vi "ref_Elbow_SEA_Oriental_position_control_frequency_lys_pwm.vi"() -> ()   [LabVIEW 2014]
uses:
  <vilib>/rvi/FXPMathLib/FxpSub/XNode/nifxpmath_Sub.xnode
  <vilib>/rvi/FXPMathLib/sim/FxpSim.dll
  <vilib>/rvi/FXPMathLib/FxpMul/XNode/nifxpmath_Multiplier.xnode
  <vilib>/rvi/FXPMathLib/FxpAdd/XNode/nifxpmath_Add.xnode
  <vilib>/eio/EIONode/EIONode.xnode
  <vilib>/rvi/eio/common/nirviEmuTemplateMethod_errors.vi
  <vilib>/rvi/FXPMathLib/FxpSinAndCos/subVIs/nifxpmath_SinAndCos_SimConfig.ctl
  <vilib>/rvi/FXPMathLib/FxpSinAndCos/simVIs/DllFxpSinAndCosTemp_sub.vi
  <vilib>/rvi/FXPMathLib/FxpSinAndCos/XNode/nifxpmath_SinAndCos.xnode
  <vilib>/rvi/Analysis/measure/butterworth/XNode/niFpgaButterworthFilter.xnode
  <vilib>/rvi/DataTransferAndStorage/Container/XNode/niFpgaContainer.xnode
  <vilib>/rvi/interface/RandomDataEmulation/nirviRandomDataFpgaMultiElementTemplate.vi
panel:
  in  "pwm method":i32
  out "tri_wave time (s)":fxp<+,64,32>
  out "vb_ pwm":fxp<+/-,21,6> format="%.21g"
  out "vb_ori":fxp<+/-,20,5> format="%.21g"
  out "va_pwm":fxp<+/-,21,6> format="%.21g"
  out "va_ori":fxp<+/-,20,5> format="%.21g"
  out "pwm_signal 2":fxp<+/-,20,5>
  in  "PWM ON":bool
  out "pwm_signal":fxp<+/-,13,6>
  out "tri_wave Ts (s)":fxp<+,37,17>=0.0009765625
  in  "Sin_magnitude_b(mm)":fxp<+/-,11,8>
  in  "Sin_offset_b (mm)":fxp<+/-,12,8>
  out "sin_signal":fxp<+/-,20,5>
  in  "Sin wave frenqueny (Hz)":fxp<+,18,3>
  out "tri_wave":fxp<+/-,64,32>
  in  "tri_wave frequency (Hz)":fxp<+,36,20>
  in  "Vdc":fxp<+,12,5>
  in  "scaled coefficients_dFb_PID":i32[](array[numeric])=[1067016412, 3362706]
  in  "Coe Ini":bool
  out "chirp_signal":fxp<+/-,36,11>
  out "frequency (Hz)":fxp<+,24,9>
  in  "Sin wave amplitude (mm)":fxp<+,20,11>
  in  "Db_step (mm)":fxp<+/-,36,11>
  in  "Step/Chirp":bool
  in  "initial frenqueny (Hz)":fxp<+,20,5>
  in  "target frenqueny (Hz)":fxp<+,23,8>
  in  "target time (s)":fxp<+,24,9>
  out "Sin wave time (s)":fxp<+,64,32>
  out "vb_b":fxp<+/-,20,5> format="%.21g"
  out "va_b":fxp<+/-,20,5> format="%.21g"
  in  "Stop Motor_b":bool
  out "dFb_PID":fxp<+/-,25,15>
  in  "dF_PID_add":bool
  out "vd_b_F":fxp<+/-,20,5>
  out "vq_b_F":fxp<+/-,20,5> format="%.57g"
  out "rad(NrTheta)_b":fxp<+/-,33,18> format="%.21g"
  out "Db(mm)":fxp<+/-,22,7>
  in  "Encoder Reset_b":bool
  in  "Db_d_M_Tc (mSec)":u32 format="%#_6f"
  out "mt_omega":u32
  in  "mt0_omega":u32
  in  "Db_M_avg_Tc (uSec)":u32
  out "Encoder Position_b":i32
  out "Omega_b(M)":fxp<+/-,32,12>
  out "Db_d(M method)":fxp<+/-,25,10>
  out "Omega_b(M_avg)":fxp<+/-,32,12>
  out "Db_d(M_avg method)":fxp<+/-,25,10>
  in  "Method case":i32
  out "Db_d(mm/s)":fxp<+/-,25,10>
  out "Omega_b(rad/s)":fxp<+/-,32,12>
  out "Omega_b(T)":fxp<+/-,20,9>
  out "Db_d(T method)":fxp<+/-,25,10>
  in  "Friction comp_b":fxp<+/-,20,10>
  out "Dbr":fxp<+/-,36,11>
  out "Dbr_d":fxp<+/-,25,15>
  out "Dbt_i":fxp<+/-,34,18>
  out "Fb_PID":fxp<+/-,22,12>
  in  "Db_tolerance":fxp<+,32,9>=1.0
  out "Db_tilde":fxp<+/-,21,11>
  in  "Kpb":fxp<+,12,8>=0.375
  in  "Kib":fxp<+,27,10>
  in  "Kdb":fxp<+,26,2>
  in  "FF or not":bool
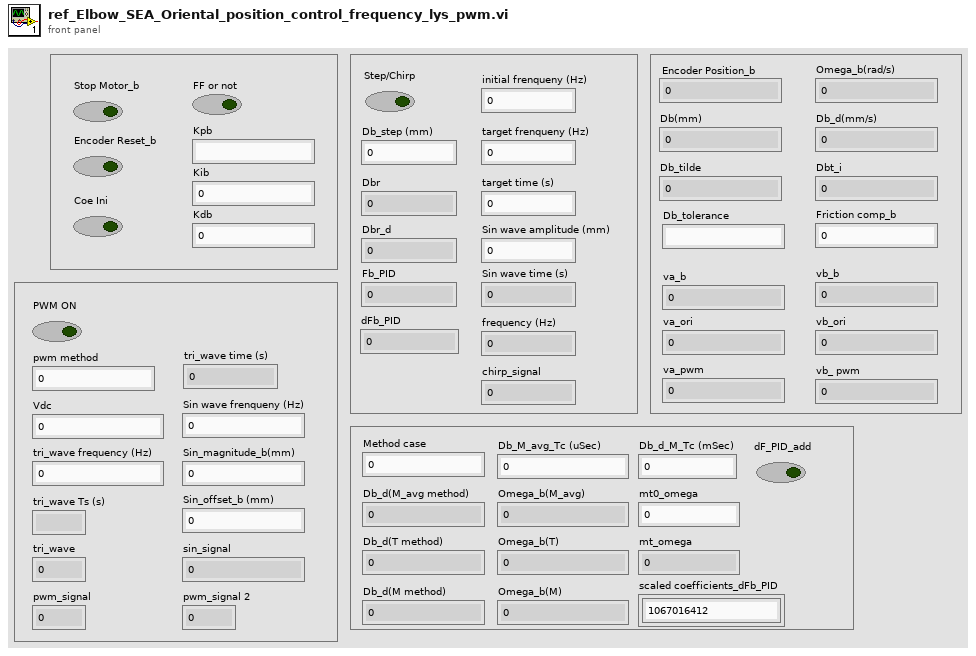
[diagram p1: front panel]
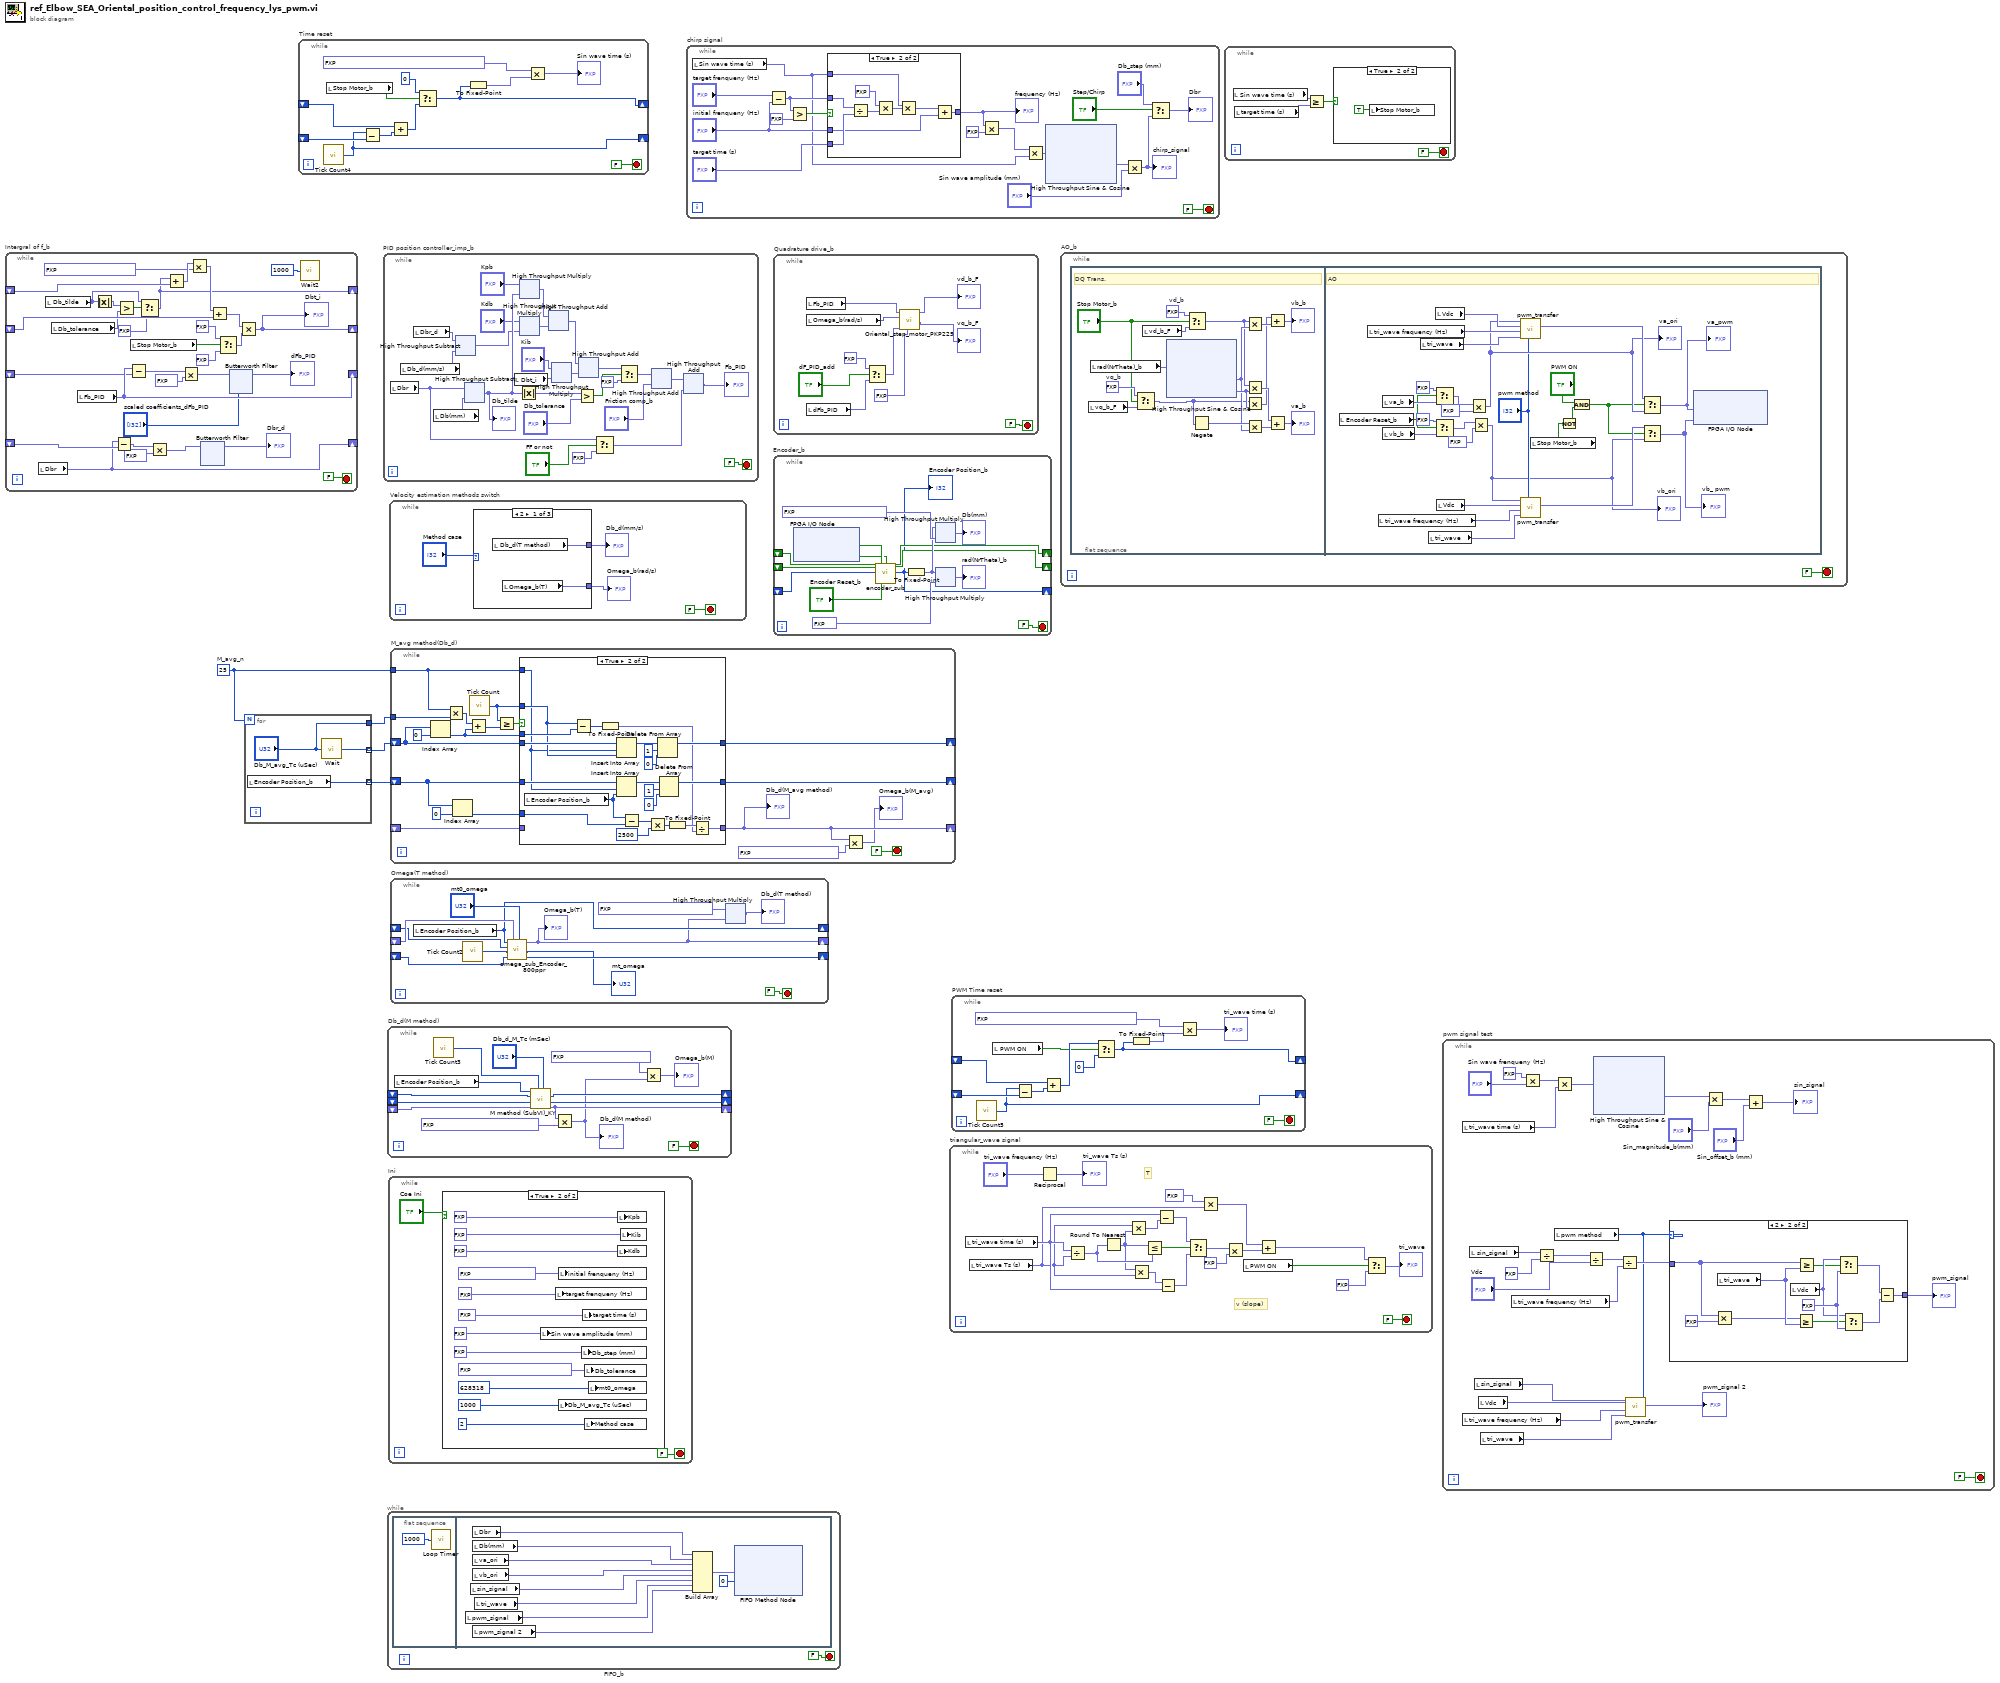
[diagram p0: block diagram]
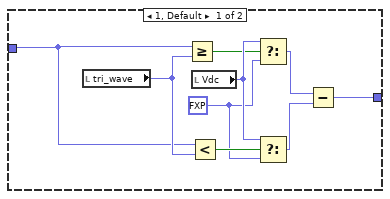
[diagram p2: hidden frame]
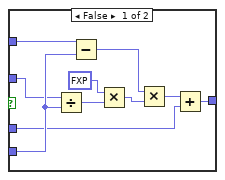
[diagram p5: hidden frame]
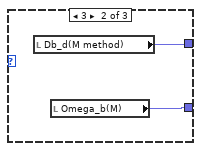
[diagram p7: hidden frame]
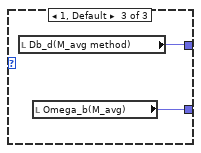
[diagram p8: hidden frame]
diagram:
  w2 = 25  # M_avg_n
  n1 = while "Intergral of f_b" {
    shift-right: [w24] -> _
    shift-left: _ -> [w25]
    shift-right: [w6] -> _
    shift-left: _ -> [w30]
    shift-right: [w20] -> _
    shift-left: _ -> [w18]
    shift-right: [w12] -> _
    shift-left: _ -> [w13]
    stop <- FALSE stop-if-true
    n2 = local read "Dbr"() -> (w12:fxp<+/-,36,11>)
    n3 = local read "Db_tilde"() -> (w26:fxp<+/-,21,11>)
    n4 = local read "Db_tolerance"() -> (w28:fxp<+,32,9>)
    n5 = local read "Fb_PID"() -> (w20:fxp<+/-,22,12>)
    n6 = Absolute Value(x=w26) -> (abs(x)=w29:fxp<+,21,11>)
    n7 = Subtract(x=w12, y=w13) -> (x-y=w15:fxp<+/-,37,12>)
    n8 = Greater?(x=w29, y=w28) -> (0:w27:bool)
    n9 = Subtract(x=w20, y=w18) -> (x-y=w19:fxp<+/-,23,13>)
    n10 = local read "Stop Motor_b"() -> (w32:bool)
    n11 = Select(t=w26, s=w27, f=fxp<+/-,21,11> 0.0) -> (s? t:f=w24:fxp<+/-,21,11>)
    n12 = Multiply(x=w15, y=fxp<+/-,24,11> 1000.0) -> (x*y=w14:fxp<+/-,25,15>)
    n13 = Add(x=w24, y=w25) -> (x+y=w34:fxp<+/-,22,12>)
    n14 = Multiply(x=w19, y=fxp<+,10,10> 1000.0) -> (x*y=w17:fxp<+/-,25,15>)
    n15 = Multiply(x=w34, y=fxp<+/-,30,12> 0.000499725341796875) -> (x*y=w31:fxp<+/-,25,15>)
    n16 = xnode "Butterworth Filter"("input data"=w14) -> ("output data"=→"Dbr_d":fxp<+/-,25,15>)  [unwired: 2 in]
    n17 = Add(x=w31, y=w30) -> (x+y=w9:fxp<+/-,32,16>)
    n18 = Select(t=fxp<+/-,2,2> 0.0, s=w32, f=fxp<+/-,2,2> 1.0) -> (s? t:f=w10:fxp<+/-,2,2>)
    n19 = xnode "Butterworth Filter"("input data"=w17, "scaled coefficients"="scaled coefficients_dFb_PID") -> ("output data"=→"dFb_PID":fxp<+/-,25,15>)  [unwired: 1 in]
    n20 = Multiply(x=w9, y=w10) -> (x*y=w6:fxp<+/-,34,18>)
    "Dbt_i" <- w6
    n21 = call "Wait2"("Count(uSec)"=u32 1000 ("Count(mSec)")) -> ()  [unwired: 1 out]
  }
  n22 = for {
    N: w2 -> [_]
    tunnel: [w55] -> w4 mode=indexing
    tunnel: [w53] -> w3 mode=indexing
    tunnel: ["Db_M_avg_Tc (uSec)"] -> w1
    n23 = local read "Encoder Position_b"() -> (w53:i32)
    n24 = call "Wait"("Count(uSec)"="Db_M_avg_Tc (uSec)") -> ("Tick Count(uSec)"=w55:u32)
  }
  n25 = while "Time reset" {
    shift-right: [w66] -> _
    shift-left: _ -> [w67]
    shift-right: [w59] -> _
    shift-left: _ -> [w61]
    stop <- FALSE stop-if-true
    n26 = call "Tick Count4"() -> ("Tick Count(uSec)"=w66:u32)
    n27 = local read "Stop Motor_b"() -> (w64:bool)
    n28 = Subtract(x=w66, y=w67) -> (x-y=w63:u32)
    n29 = Add(x=w61, y=w63) -> (x+y=w62:u32)
    n30 = Select(t=u32 0, s=w64, f=w62) -> (s? t:f=w59:u32)
    n31 = To Fixed-Point(number=w59) -> (fixed-point=w57:fxp<+,64,32>)  [unwired: 1 in]
    n32 = Multiply(x=fxp<+,20,-18> 1.0000003385357559e-06 ("y"), y=w57) -> (x*y=→"Sin wave time (s)":fxp<+,64,32>)
  }
  n33 = while "PID position controller_imp_b" {
    stop <- FALSE stop-if-true
    n34 = local read "Dbr"() -> (w69:fxp<+/-,36,11>)
    n35 = local read "Db_d(mm/s)"() -> (w76:fxp<+/-,25,10>)
    n36 = local read "Dbr_d"() -> (w75:fxp<+/-,25,15>)
    n37 = local read "Db(mm)"() -> (w87:fxp<+/-,22,7>)
    n38 = xnode "High Throughput Subtract"("x"=w75, "y"=w76) -> ("x-y"=w77:fxp<+/-,31,16>)
    n39 = xnode "High Throughput Subtract"("x"=w69, "y"=w87) -> ("x-y"=w89:fxp<+/-,21,11>)
    "Db_tilde" <- w89
    n40 = local read "Dbt_i"() -> (w85:fxp<+/-,34,18>)
    n41 = Absolute Value(x=w89) -> (abs(x)=w92:fxp<+,21,11>)
    n42 = xnode ("High Throughput Multiply")("x"="Kpb", "y"=w89) -> ("x*y"=w88:fxp<+/-,33,17>)
    n43 = xnode ("High Throughput Multiply")("x"="Kdb", "y"=w77) -> ("x*y"=w82:fxp<+/-,31,21>)
    n44 = xnode ("High Throughput Add")("x"=w88, "y"=w82) -> ("x+y"=w86:fxp<+/-,22,12>)
    n45 = xnode ("High Throughput Multiply")("x"="Kib", "y"=w85) -> ("x*y"=w84:fxp<+/-,31,14>)
    n46 = Greater?(x=w92, y="Db_tolerance") -> (0:w91:bool)
    n47 = xnode ("High Throughput Add")("x"=w86, "y"=w84) -> ("x+y"=w83:fxp<+/-,22,12>)
    n48 = Select(t=w69, s="FF or not", f=fxp<+/-,36,11> 0.0) -> (s? t:f=w71:fxp<+/-,36,11>)
    n49 = Select(t=w83, s=w91, f=fxp<+/-,20,10> 0.0) -> (s? t:f=w81:fxp<+/-,22,12>)
    n50 = xnode ("High Throughput Add")("x"=w81, "y"="Friction comp_b") -> ("x+y"=w73:fxp<+/-,22,12>)
    n51 = xnode ("High Throughput Add")("x"=w73, "y"=w71) -> ("x+y"=→"Fb_PID":fxp<+/-,22,12>)
  }
  n52 = while "Db_d(M method)" {
    shift-right: [w106] -> _
    shift-left: _ -> [w101]
    shift-right: [w105] -> _
    shift-left: _ -> [w100]
    shift-right: [w98] -> _
    shift-left: _ -> [w99]
    stop <- FALSE stop-if-true
    n53 = local read "Encoder Position_b"() -> (w102:i32)
    n54 = call "Tick Count3"() -> ("Tick Count(mSec)"=w103:u32)
    n55 = call "M method (SubVI)_KY.vi"("Tc (mSec)"="Db_d_M_Tc (mSec)", "Tick Count (mSec)"=w103, "Encoder velocity_pre (pulse/s)"=w99, "Shift Register in 2"=w100, "Shift Register in 1"=w101, "Encoder pulses"=w102) -> ("Encoder velocity (pulse/s)"=w98:fxp<+/-,64,32>, "Shift Register out 2"=w105:i32, "Shift Register out 1"=w106:u32)  [unwired: 3 in]
    n56 = Multiply(x=w98, y=fxp<+/-,20,-5> 0.002499997615814209) -> (x*y=w95:fxp<+/-,25,10>)
    "Db_d(M method)" <- w95
    n57 = Multiply(x=fxp<+/-,32,12> 3.1415929794311523, y=w95) -> (x*y=→"Omega_b(M)":fxp<+/-,32,12>)
  }
  n58 = while "FIFO_b" {
    stop <- FALSE stop-if-true
    n59 = flat-sequence {
      frame #0 {
        n60 = call "Loop Timer"("Count(uSec)"=u32 1000 ("Loop Period (usec)")) -> ()  [unwired: 1 out]
      }
      frame #1 {
        n61 = local read "pwm_signal"() -> (w113:fxp<+/-,13,6>)
        n62 = local read "sin_signal"() -> (w114:fxp<+/-,20,5>)
        n63 = local read "Dbr"() -> (w117:fxp<+/-,36,11>)
        n64 = local read "Db(mm)"() -> (w116:fxp<+/-,22,7>)
        n65 = local read "va_ori"() -> (w115:fxp<+/-,20,5>)
        n66 = local read "vb_ori"() -> (w120:fxp<+/-,20,5>)
        n67 = local read "pwm_signal 2"() -> (w119:fxp<+/-,20,5>)
        n68 = local read "tri_wave"() -> (w112:fxp<+/-,64,32>)
        n69 = Build Array(w117, w116, w115, w120, w114, w112, w113, w119) -> (w111:fxp<+/-,64,32>[])
        n70 = xnode ("FIFO Method Node")("Element"=w111, "Timeout"=0) -> ()  [unwired: 1 in, 2 out]
      }
    }
  }
  n71 = while "Ini" {
    stop <- FALSE stop-if-true
    n72 = case shown="True" "Coe Ini" {
      frame False {
      }
      frame True {
        n73 = local write "Sin wave amplitude (mm)"(fxp<+,20,11> 0.0 ("target frenqueny (Hz)")) -> ()
        n74 = local write "target frenqueny (Hz)"(fxp<+,23,8> 10.0 ("target frenqueny (Hz)")) -> ()
        n75 = local write "initial frenqueny (Hz)"(fxp<+,20,5> 0.100006103515625 ("initial frenqueny (Hz)")) -> ()
        n76 = local write "Db_M_avg_Tc (uSec)"(u32 1000 ("M_avg_Tc (uSec)")) -> ()
        n77 = local write "Db_step (mm)"(fxp<+/-,36,11> 0.0 ("target frenqueny (Hz)")) -> ()
        n78 = local write "target time (s)"(fxp<+,24,9> 120.0 ("target time (s)")) -> ()
        n79 = local write "Db_tolerance"(fxp<+,32,9> 0.10000002384185791) -> ()
        n80 = local write "Method case"(2 ("M_avg_Tc (uSec)")) -> ()
        n81 = local write "mt0_omega"(u32 628318 ("mt0_omega")) -> ()
        n82 = local write "Kpb"(fxp<+,11,7> 0.0) -> ()
        n83 = local write "Kdb"(fxp<+,26,2> 0.0) -> ()
        n84 = local write "Kib"(fxp<+,27,10> 0.0 ("Kiy 2")) -> ()
      }
    }
  }
  n85 = while "Velocity estimation methods switch" {
    stop <- FALSE stop-if-true
    n86 = case shown="2" "Method case" {
      tunnel: [w139 w141 w143] -> w136
      tunnel: [w140 w142 w144] -> w135
      frame 2 {
        n87 = local read "Db_d(T method)"() -> (w139:fxp<+/-,25,10>)
        n88 = local read "Omega_b(T)"() -> (w140:fxp<+/-,20,9>)
      }
      frame 3 {
        n89 = local read "Db_d(M method)"() -> (w141:fxp<+/-,25,10>)
        n90 = local read "Omega_b(M)"() -> (w142:fxp<+/-,32,12>)
      }
      frame 1, Default {
        n91 = local read "Db_d(M_avg method)"() -> (w143:fxp<+/-,25,10>)
        n92 = local read "Omega_b(M_avg)"() -> (w144:fxp<+/-,32,12>)
      }
    }
    "Db_d(mm/s)" <- w136
    "Omega_b(rad/s)" <- w135
  }
  n93 = while "M_avg method(Db_d)" {
    shift-right: [w155] -> _
    shift-left: w4 -> [w158]
    tunnel: w2 -> [w156]
    shift-right: [w153] -> _
    shift-left: w3 -> [w151]
    shift-right: [w146] -> _
    shift-left: _ -> [w149]
    tunnel: w1 -> [w148]
    stop <- FALSE stop-if-true
    n94 = Index Array(array=w158, index=0) -> (element=w154:u32)
    n95 = Multiply(x=w156, y=w148) -> (x*y=w161:u32)
    n96 = Index Array(array=w151, index=0) -> (element=w150:i32)
    n97 = Add(x=w161, y=w154) -> (x+y=w160:u32)
    n98 = call "Tick Count"() -> ("Tick Count(uSec)"=w157:u32)
    n99 = Greater Or Equal?(x=w157, y=w160) -> (x >= y?=w159:bool)
    n100 = case shown="True" w159 {
      tunnel: w158 -> [w166 w188]
      tunnel: w157 -> [_ w182]
      tunnel: w156 -> [_ w171]
      tunnel: [w166 w184] -> w155
      tunnel: w154 -> [_ w183]
      tunnel: w151 -> [w165 w172]
      tunnel: [w165 w170] -> w153
      tunnel: [w164 w169] -> w146
      tunnel: w150 -> [_ w167]
      tunnel: w149 -> [w164 _]
      frame False {
      }
      frame True {
        n101 = local read "Encoder Position_b"() -> (w176:i32)
        n102 = Subtract(x=w182, y=w183) -> (x-y=w181:u32)
        n103 = To Fixed-Point(number=w181) -> (fixed-point=w168:fxp<+,32,32>)  [unwired: 1 in]
        n104 = Insert Into Array(array=w188, index=w171, new element=w182) -> (w187:u32[])
        n105 = Insert Into Array(array=w172, index=w171, new element=w176) -> (w173:i32[])
        n106 = Subtract(x=w176, y=w167) -> (x-y=w177:i32)
        n107 = Multiply(x=w177, y=2500) -> (x*y=w179:i32)
        n108 = Delete From Array(array=w187, length=1, index=0) -> (array with subset deleted=w184:u32[])  [unwired: 1 out]
        n109 = Delete From Array(array=w173, length=1, index=0) -> (array with subset deleted=w170:i32[])  [unwired: 1 out]
        n110 = To Fixed-Point(number=w179) -> (fixed-point=w180:fxp<+/-,32,32>)  [unwired: 1 in]
        n111 = Divide(x=w180, y=w168) -> (x/y=w169:fxp<+/-,25,10>)
      }
    }
    "Db_d(M_avg method)" <- w146
    n112 = Multiply(x=w146, y=fxp<+/-,32,12> 3.1415929794311523 ("x")) -> (x*y=→"Omega_b(M_avg)":fxp<+/-,32,12>)
  }
  n113 = while "Omega(T method)" {
    shift-right: [w193] -> _
    shift-left: _ -> [w192]
    shift-right: [w199] -> _
    shift-left: _ -> [w194]
    shift-right: [w190] -> _
    shift-left: _ -> [w196]
    stop <- FALSE stop-if-true
    n114 = local read "Encoder Position_b"() -> (w193:i32)
    n115 = call "Tick Count2"() -> ("Tick Count(Ticks)"=w195:u32)
    n116 = call "omega_sub_Encoder_800ppr.vi"("mt0"="mt0_omega", "omega_pre"=w196, "ticks_m_pre"=w194, "ticks"=w195, "count_pre"=w192, "count"=w193) -> ("ticks_m"=w199:u32, "mt"=→"mt_omega":u32, "omega"=w190:fxp<+/-,20,9>)  [unwired: 3 in]
    "Omega_b(T)" <- w190
    n117 = xnode ("High Throughput Multiply")("x"=fxp<+/-,26,1> 0.3183099031448364, "y"=w190) -> ("x*y"=→"Db_d(T method)":fxp<+/-,24,9>)
  }
  n118 = while "chirp signal" {
    stop <- FALSE stop-if-true
    n119 = local read "Sin wave time (s)"() -> (w202:fxp<+,64,32>)
    n120 = Subtract(x="target frenqueny (Hz)", y="initial frenqueny (Hz)") -> (x-y=w203:fxp<+/-,24,9>)
    n121 = Greater?(x=w203, y=fxp<+/-,24,9> 0.0) -> (0:w206:bool)
    n122 = case shown="True" w206 {
      tunnel: [w227 w236] -> w211
      tunnel: "target time (s)" -> [w224 w235]
      tunnel: "initial frenqueny (Hz)" -> [w223 w234]
      tunnel: w202 -> [w226 w233]
      tunnel: w203 -> [w222 w232]
      frame False {
        n123 = Divide(x=w222, y=w224) -> (x/y=w221:fxp<+/-,24,9>)
        n124 = Subtract(x=w226, y=w224) -> (x-y=w225:fxp<+/-,24,9>)
        n125 = Multiply(x=fxp<+/-,24,9> 0.5, y=w221) -> (x*y=w220:fxp<+/-,23,10>)
        n126 = Multiply(x=w225, y=w220) -> (x*y=w228:fxp<+/-,26,11>)
        n127 = Add(x=w228, y=w223) -> (x+y=w227:fxp<+,24,9>)
      }
      frame True {
        n128 = Divide(x=w232, y=w235) -> (x/y=w230:fxp<+/-,24,9>)
        n129 = Multiply(x=fxp<+/-,24,9> 0.5, y=w230) -> (x*y=w231:fxp<+/-,23,10>)
        n130 = Multiply(x=w233, y=w231) -> (x*y=w237:fxp<+/-,26,11>)
        n131 = Add(x=w237, y=w234) -> (x+y=w236:fxp<+,24,9>)
      }
    }
    "frequency (Hz)" <- w211
    n132 = Multiply(x=w211, y=fxp<+,1,2> 2.0) -> (x*y=w217:fxp<+,25,10>)
    n133 = Multiply(x=w217, y=w202) -> (x*y=w210:fxp<+,33,18>)
    n134 = xnode "High Throughput Sine & Cosine"("x (pi)"=w210) -> ("sin(x)"=w209:fxp<+/-,16,2>)  [unwired: 1 out]
    n135 = Multiply(x=w209, y="Sin wave amplitude (mm)") -> (x*y=w214:fxp<+/-,36,11>)
    "chirp_signal" <- w214
    n136 = Select(t="Db_step (mm)", s="Step/Chirp", f=w214) -> (s? t:f=→"Dbr":fxp<+/-,36,11>)
  }
  n137 = while "Encoder_b" {
    shift-right: [w270] -> _
    shift-left: _ -> [w281]
    shift-right: [w269] -> _
    shift-left: _ -> [w280]
    shift-right: [w268] -> _
    shift-left: _ -> [w279]
    stop <- FALSE stop-if-true
    n138 = xnode "FPGA I/O Node"() -> ("Mod4/DI3"=w272:bool, "Mod4/DI4"=w271:bool)  [unwired: 2 in, 2 out]
    n139 = call "encoder_sub.vi"("A_pre"=w281, "B_pre"=w280, "Encoder Position_pre"=w279, "A input"=w272, "Encoder Position Reset"="Encoder Reset_b", "B input"=w271) -> ("A"=w270:bool, "B"=w269:bool, "Encoder Position (Counts)"=w268:i32)  [unwired: 19 in]
    "Encoder Position_b" <- w268
    n140 = To Fixed-Point(number=w268) -> (fixed-point=w276:fxp<+/-,18,18>)  [unwired: 1 in]
    n141 = xnode ("High Throughput Multiply")("x"=w276, "y"=fxp<+/-,15,-7> 0.0025000572204589844) -> ("x*y"=→"Db(mm)":fxp<+/-,22,7>)
    n142 = xnode ("High Throughput Multiply")("x"=w276, "y"=fxp<+,24,0> 0.125) -> ("x*y"=→"rad(NrTheta)_b":fxp<+/-,33,18>)
  }
  n143 = while "Quadrature drive_b" {
    stop <- FALSE stop-if-true
    n144 = local read "Fb_PID"() -> (w286:fxp<+/-,22,12>)
    n145 = local read "Omega_b(rad/s)"() -> (w285:fxp<+/-,32,12>)
    n146 = local read "dFb_PID"() -> (w289:fxp<+/-,25,15>)
    n147 = Select(t=fxp<+/-,25,15> 0.0 ("f"), s="dF_PID_add", f=w289) -> (s? t:f=w284:fxp<+/-,25,15>)
    n148 = call "Oriental_step_motor_PKP225.vi"("F_Threshold"=fxp<+,12,12> 10.0, "dFmr"=w284, "omega"=w285, "Fmr"=w286) -> ("vq_F"=→"vq_b_F":fxp<+/-,20,5>, "vd_F"=→"vd_b_F":fxp<+/-,20,5>)  [unwired: 6 in]
  }
  n149 = while "triangular_wave signal" {
    stop <- FALSE stop-if-true
    # "T"
    # "v (slope)"
    n150 = local read "tri_wave time (s)"() -> (w303:fxp<+,64,32>)
    n151 = local read "tri_wave Ts (s)"() -> (w299:fxp<+,37,17>)
    n152 = Reciprocal(x="tri_wave frequency (Hz)") -> (1/x=→"tri_wave Ts (s)":fxp<+,37,17>)
    n153 = Divide(x=w303, y=w299) -> (x/y=w304:fxp<+,64,53>)
    n154 = Round To Nearest(number=w304) -> (nearest integer value=w301:fxp<+,54,54>)
    n155 = Multiply(x=w299, y=w301) -> (x*y=w302:fxp<+,64,32>)
    n156 = Multiply(x=w301, y=w299) -> (x*y=w300:fxp<+,64,32>)
    n157 = Less Or Equal?(x=w301, y=w304) -> (x <= y?=w311:bool)
    n158 = Subtract(x=w303, y=w302) -> (x-y=w308:fxp<+/-,64,32>)
    n159 = Subtract(x=w300, y=w303) -> (x-y=w307:fxp<+/-,64,32>)
    n160 = Select(t=w308, s=w311, f=w307) -> (s? t:f=w306:fxp<+/-,64,32>)
    n161 = Multiply(x=fxp<+/-,1,0> -0.5, y=w299) -> (x*y=w309:fxp<+/-,38,17>)
    n162 = Multiply(x=w306, y=fxp<+,1,2> 2.0) -> (x*y=w305:fxp<+/-,64,32>)
    n163 = local read "PWM ON"() -> (w294:bool)
    n164 = Add(x=w309, y=w305) -> (x+y=w297:fxp<+/-,64,32>)
    n165 = Select(t=w297, s=w294, f=fxp<+,1,1> 0.0) -> (s? t:f=→"tri_wave":fxp<+/-,64,32>)
  }
  n166 = while "PWM Time reset" {
    shift-right: [w324] -> _
    shift-left: _ -> [w325]
    shift-right: [w320] -> _
    shift-left: _ -> [w321]
    stop <- FALSE stop-if-true
    n167 = call "Tick Count5"() -> ("Tick Count(uSec)"=w324:u32)
    n168 = local read "PWM ON"() -> (w314:bool)
    n169 = Subtract(x=w324, y=w325) -> (x-y=w322:u32)
    n170 = Add(x=w321, y=w322) -> (x+y=w316:u32)
    n171 = Select(t=w316, s=w314, f=u32 0 ("t")) -> (s? t:f=w320:u32)
    n172 = To Fixed-Point(number=w320) -> (fixed-point=w318:fxp<+,64,32>)  [unwired: 1 in]
    n173 = Multiply(x=fxp<+,20,-18> 1.0000003385357559e-06 ("y"), y=w318) -> (x*y=→"tri_wave time (s)":fxp<+,64,32>)
  }
  n174 = while "AO_b" {
    stop <- FALSE stop-if-true
    n175 = flat-sequence {
      frame #0 {
        w333 = fxp<+/-,20,5> 0.0  # vq_b
        w332 = fxp<+/-,20,5> 0.0  # vd_b
        # "DQ Trans."
        n176 = local read "vq_b_F"() -> (w330:fxp<+/-,20,5>)
        n177 = local read "rad(NrTheta)_b"() -> (w343:fxp<+/-,33,18>)
        n178 = Select(t=w333, s="Stop Motor_b", f=w330) -> (s? t:f=w327:fxp<+/-,20,5>)
        n179 = local read "vd_b_F"() -> (w331:fxp<+/-,20,5>)
        n180 = xnode "High Throughput Sine & Cosine"("x (pi)"=w343) -> ("sin(x)"=w334:fxp<+/-,17,2>, "cos(x)"=w335:fxp<+/-,17,2>)
        n181 = Select(t=w332, s="Stop Motor_b", f=w331) -> (s? t:f=w328:fxp<+/-,20,5>)
        n182 = Negate(x=w327) -> (-x=w342:fxp<+/-,21,6>)
        n183 = Multiply(x=w328, y=w334) -> (x*y=w338:fxp<+/-,20,5>)
        n184 = Multiply(x=w328, y=w335) -> (x*y=w341:fxp<+/-,20,5>)
        n185 = Multiply(x=w327, y=w335) -> (x*y=w337:fxp<+/-,20,5>)
        n186 = Multiply(x=w342, y=w334) -> (x*y=w340:fxp<+/-,20,5>)
        n187 = Add(x=w337, y=w338) -> (x+y=→"vb_b":fxp<+/-,20,5>)
        n188 = Add(x=w341, y=w340) -> (x+y=→"va_b":fxp<+/-,20,5>)
      }
      frame #1 {
        # "AO"
        n189 = local read "Encoder Reset_b"() -> (w395:bool)
        n190 = local read "tri_wave frequency (Hz)"() -> (w386:fxp<+,36,20>)
        n191 = local read "tri_wave frequency (Hz)"() -> (w389:fxp<+,36,20>)
        n192 = local read "va_b"() -> (w396:fxp<+/-,20,5>)
        n193 = local read "vb_b"() -> (w397:fxp<+/-,20,5>)
        n194 = local read "tri_wave"() -> (w385:fxp<+/-,64,32>)
        n195 = local read "tri_wave"() -> (w388:fxp<+/-,64,32>)
        n196 = Select(t=fxp<+/-,20,5> 3.0 ("Mod2/AO4"), s=w395, f=w396) -> (s? t:f=w394:fxp<+/-,20,5>)
        n197 = Select(t=fxp<+/-,20,5> 0.0 ("Mod2/AO4"), s=w395, f=w397) -> (s? t:f=w391:fxp<+/-,20,5>)
        n198 = local read "Vdc"() -> (w384:fxp<+,12,5>)
        n199 = local read "Vdc"() -> (w390:fxp<+,12,5>)
        n200 = Multiply(x=w394, y=fxp<+/-,20,5> -0.5) -> (x*y=w382:fxp<+/-,20,5>)
        "va_ori" <- w382
        n201 = Multiply(x=w391, y=fxp<+/-,20,5> -0.5) -> (x*y=w376:fxp<+/-,20,5>)
        "vb_ori" <- w376
        n202 = call "pwm_transfer.vi"("pwm method"="pwm method", "tri_wave"=w385, "tri_wave frequency (Hz)"=w386, "Vdc"=w384, "signal_input"=w382) -> ("pwm_signal"=w383:fxp<+/-,20,5>)  [unwired: 6 in]
        n203 = call "pwm_transfer.vi"("pwm method"="pwm method", "tri_wave"=w388, "tri_wave frequency (Hz)"=w389, "Vdc"=w390, "signal_input"=w376) -> ("pwm_signal"=w387:fxp<+/-,20,5>)  [unwired: 6 in]
        n204 = local read "Stop Motor_b"() -> (w378:bool)
        n205 = Not(x=w378) -> (.not. x?=w377:bool)
        n206 = And(x="PWM ON", y=w377) -> (x .and. y?=w380:bool)
        n207 = Select(t=w383, s=w380, f=w382) -> (s? t:f=w374:fxp<+/-,20,5>)
        "va_pwm" <- w374
        n208 = Select(t=w387, s=w380, f=w376) -> (s? t:f=w375:fxp<+/-,20,5>)
        "vb_ pwm" <- w375
        n209 = xnode "FPGA I/O Node"("Mod8/AO14"=w374, "Mod8/AO15"=w375) -> ()  [unwired: 2 in, 2 out]
      }
    }
  }
  n210 = while {
    stop <- FALSE stop-if-true
    n211 = local read "Sin wave time (s)"() -> (w402:fxp<+,64,32>)
    n212 = local read "target time (s)"() -> (w401:fxp<+,24,9>)
    n213 = Greater Or Equal?(x=w402, y=w401) -> (x >= y?=w400:bool)
    n214 = case shown="True" w400 {
      frame False {
      }
      frame True {
        n215 = local write "Stop Motor_b"(TRUE ("Stop Motor_b")) -> ()
      }
    }
  }
  n216 = while "pwm signal test" {
    stop <- FALSE stop-if-true
    n217 = local read "tri_wave time (s)"() -> (w418:fxp<+,64,32>)
    n218 = local read "tri_wave frequency (Hz)"() -> (w427:fxp<+,36,20>)
    n219 = local read "sin_signal"() -> (w409:fxp<+/-,20,5>)
    n220 = local read "sin_signal"() -> (w425:fxp<+/-,20,5>)
    n221 = local read "Vdc"() -> (w426:fxp<+,12,5>)
    n222 = local read "tri_wave"() -> (w428:fxp<+/-,64,32>)
    n223 = local read "tri_wave frequency (Hz)"() -> (w414:fxp<+,36,20>)
    n224 = Multiply(x=fxp<+,1,2> 2.0 ("y"), y="Sin wave frenqueny (Hz)") -> (x*y=w417:fxp<+/-,20,6>)
    n225 = Divide(x=w409, y=fxp<+,1,2> 2.0) -> (x/y=w411:fxp<+/-,21,4>)
    n226 = Multiply(x=w417, y=w418) -> (x*y=w419:fxp<+/-,48,18>)
    n227 = local read "pwm method"() -> (w405:i32)
    n228 = Divide(x=w411, y="Vdc") -> (x/y=w413:fxp<+/-,33,11>)
    n229 = xnode "High Throughput Sine & Cosine"("x (pi)"=w419) -> ("sin(x)"=w424:fxp<+/-,17,2>)  [unwired: 1 out]
    n230 = Divide(x=w413, y=w414) -> (x/y=w407:fxp<+/-,64,32>)
    n231 = call "pwm_transfer.vi"("pwm method"=w405, "tri_wave"=w428, "tri_wave frequency (Hz)"=w427, "Vdc"=w426, "signal_input"=w425) -> ("pwm_signal"=→"pwm_signal 2":fxp<+/-,20,5>)  [unwired: 6 in]
    n232 = case shown="2" w405 {
      tunnel: w407 -> [w431 w440]
      tunnel: [w430 w439] -> w406
      frame 1, Default {
        w432 = fxp<+,12,5> 0.0
        n233 = local read "tri_wave"() -> (w435:fxp<+/-,64,32>)
        n234 = Greater Or Equal?(x=w431, y=w435) -> (x >= y?=w433:bool)
        n235 = Less?(x=w431, y=w435) -> (x < y?=w434:bool)
        n236 = local read "Vdc"() -> (w438:fxp<+,12,5>)
        n237 = Select(t=w438, s=w433, f=w432) -> (s? t:f=w437:fxp<+,12,5>)
        n238 = Select(t=w438, s=w434, f=w432) -> (s? t:f=w436:fxp<+,12,5>)
        n239 = Subtract(x=w437, y=w436) -> (x-y=w430:fxp<+/-,13,6>)
      }
      frame 2 {
        w447 = fxp<+,12,5> 0.0
        n240 = Multiply(x=w440, y=fxp<+/-,1,1> -1.0) -> (x*y=w443:fxp<+/-,64,34>)
        n241 = local read "tri_wave"() -> (w444:fxp<+/-,64,32>)
        n242 = local read "Vdc"() -> (w446:fxp<+,12,5>)
        n243 = Greater Or Equal?(x=w443, y=w444) -> (x >= y?=w445:bool)
        n244 = Greater Or Equal?(x=w440, y=w444) -> (x >= y?=w441:bool)
        n245 = Select(t=w446, s=w441, f=w447) -> (s? t:f=w448:fxp<+,12,5>)
        n246 = Select(t=w446, s=w445, f=w447) -> (s? t:f=w449:fxp<+,12,5>)
        n247 = Subtract(x=w448, y=w449) -> (x-y=w439:fxp<+/-,13,6>)
      }
    }
    "pwm_signal" <- w406
    n248 = Multiply(x=w424, y="Sin_magnitude_b(mm)") -> (x*y=w420:fxp<+/-,20,8>)
    n249 = Add(x=w420, y="Sin_offset_b (mm)") -> (x+y=→"sin_signal":fxp<+/-,20,5>)
  }
